vi "JsonToSteps.vi"(8 "error in":errorcluster, 11 "JSON String":string) -> (0 "error out":errorcluster, 2 "All items found?":bool, 3 "Steps":refnum<class "Step.lvclass">[](array[class]))   [LabVIEW 2023, in "Easy.SequenceManagerLabVIEW.lvlib" / "Step.lvclass"]
uses:
  Step.lvclass
  6cf8f237-96dc-4f1f-a660-aec153e8deb5.vi
  054594f7-ea92-4a54-9fad-94293ff1125a.vi
  ec343c40-536c-461c-8d01-e8b2dd1d68f3.vi
  695f3286-a13c-467f-b6c6-973f5bd1729f.vi
  <vilib>/JDP Science/JSONtext/Find Item.vi
  <vilib>/JDP Science/JSONtext/Next JSON Value.vi
  <vilib>/JDP Science/JSONtext/String Subset.vi
  <vilib>/JDP Science/JSONtext/Parsing/Advance past next JSON Value (inlined COPY).vi
  <vilib>/JDP Science/JSONtext/Parsing/Advance past whitespace.vi
  <vilib>/JDP Science/JSONtext/Parsing/Advance past String.vi
  <vilib>/JDP Science/JSONtext/Parsing/Advance past Number.vi
  <vilib>/JDP Science/JSONtext/Parsing/Advance past Line Ending.vi
  <vilib>/JDP Science/JSONtext/Parsing/Parse Full Path or Item Name.vi
  <vilib>/JDP Science/JSONtext/Parsing/Advance past Array.vi
  <vilib>/JDP Science/JSONtext/Parsing/Advance past Object.vi
  <vilib>/JDP Science/JSONtext/support/Error Cluster From Code.vi
  <vilib>/JDP Science/JSONtext/Offset/Find Item Locations by Path.vi
  <vilib>/JDP Science/JSONtext/JSON text to Variant.vi
  <vilib>/JDP Science/JSONtext/LVClass Serializer/JSONtext LVClass Serializer.lvclass
  <vilib>/JDP Science/JSONtext/JSONtext.lvlib
  Parameter/Parameter.lvclass
panel:
  # "Connector Pane"
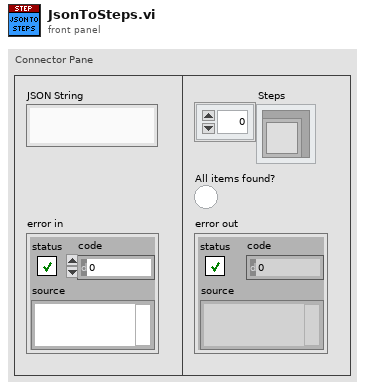
[diagram p1: front panel]
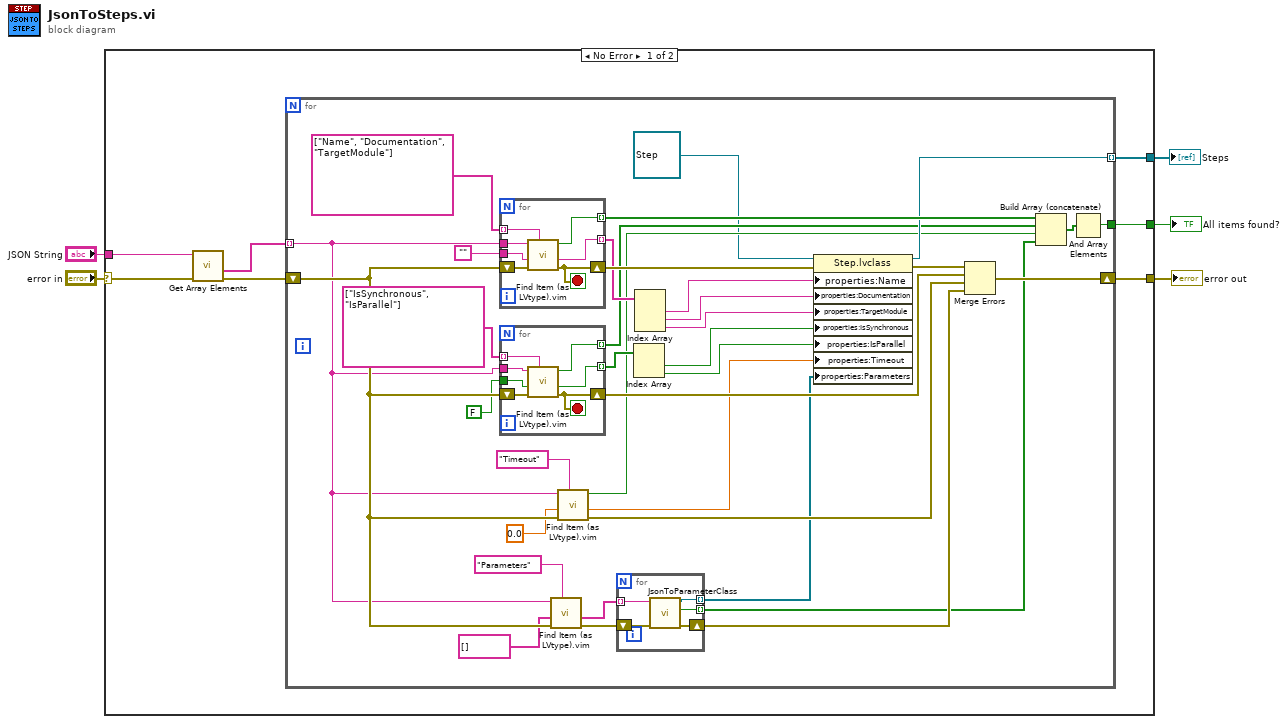
[diagram p0: block diagram]
diagram:
  n1 = case shown="No Error" "error in" {
    selector: "error in" -> [w12 w67]
    tunnel: [w10 w67] -> w4
    tunnel: "JSON String" -> [w9 _]
    tunnel: [w7 _] -> w2
    tunnel: [w6 _] -> w1
    frame No Error {
      n2 = call <vilib>:"Get Array Elements.vi"("error in (no error)"=w12, "JSON"=w9) -> ("error out"=w11:errorcluster, "<JSON>"=w8:string[])  [unwired: 7 in, 1 out]
      n3 = for {
        tunnel: w8 -> [w22] mode=indexing
        tunnel: [w18] -> w7 mode=indexing
        shift-right: [w40] -> w10
        shift-left: w11 -> [w44]
        tunnel: [w15] -> w6
        n4 = for {
          tunnel: string[] ["Name", "Documentation", "TargetModule"] -> [w64] mode=indexing
          tunnel: "" -> [w63]
          tunnel: w22 -> [w62]
          shift-right: [w65] -> w47
          shift-left: w44 -> [w66]
          tunnel: [w61] -> w35 mode=indexing
          tunnel: [w60] -> w37 mode=indexing
          stop <- w65 stop-if-true
          n5 = call "Find Item (as LVtype).vim"("$Path or Item Name"=w64, "error in (no error)"=w66, "Data Type and Default Value"=w63, "JSON"=w62) -> ("error out"=w65:errorcluster, "Data"=w61:string, "Found"=w60:bool)  [unwired: 4 in, 1 out]
        }
        n6 = for {
          tunnel: string[] ["IsSynchronous", "IsParallel"] -> [w57] mode=indexing
          tunnel: FALSE -> [w56]
          tunnel: w22 -> [w55]
          shift-right: [w58] -> w43
          shift-left: w44 -> [w59]
          tunnel: [w54] -> w29 mode=indexing
          tunnel: [w53] -> w17 mode=indexing
          stop <- w58 stop-if-true
          n7 = call "Find Item (as LVtype).vim"("$Path or Item Name"=w57, "error in (no error)"=w59, "Data Type and Default Value"=w56, "JSON"=w55) -> ("error out"=w58:errorcluster, "Data"=w54:bool, "Found"=w53:bool)  [unwired: 4 in, 1 out]
        }
        n8 = call "Find Item (as LVtype).vim"("$Path or Item Name"="Parameters", "error in (no error)"=w44, "Data Type and Default Value"=string[] [], "JSON"=w22) -> ("error out"=w46:errorcluster, "Data"=w20:string[])  [unwired: 4 in, 2 out]
        n9 = call "Find Item (as LVtype).vim"("$Path or Item Name"="Timeout", "error in (no error)"=w44, "Data Type and Default Value"=0.0, "JSON"=w22) -> ("error out"=w42:errorcluster, "Data"=w24:dbl, "Found"=w16:bool)  [unwired: 4 in, 1 out]
        n10 = for {
          tunnel: w20 -> [w50] mode=indexing
          tunnel: [w49] -> w14 mode=indexing
          tunnel: [w48] -> w19 mode=indexing
          shift-right: [w51] -> w41
          shift-left: w46 -> [w52]
          n11 = call "JsonToParameterClass.vi"("error in"=w52, "JSON String"=w50) -> ("error out"=w51:errorcluster, "All items found?"=w49:bool, "Parameter Out"=w48:refnum<class "Parameter.lvclass">)  [unwired: 7 in]
        }
        n12 = Index Array(array=w29) -> (element #1=w28:bool, element #2=w27:bool)  [unwired: 2 in]
        n13 = Index Array(array=w35) -> (element #1=w34:string, element #2=w33:string, element #3=w32:string)  [unwired: 3 in]
        n14 = property class="Step.lvclass"(reference=refnum<class "Step.lvclass"> refnum ("Easy.SequenceManagerLabVIEW.lvlib:Step.lvclass"), error in=w47, "properties:Name"=w34, "properties:Documentation"=w33, "properties:TargetModule"=w32, "properties:IsSynchronous"=w28, "properties:IsParallel"=w27, "properties:Timeout"=w24, "properties:Parameters"=w19) -> (reference out=w18:refnum<class "Step.lvclass">, error out=w45:errorcluster)
        n15 = Merge Errors(w45, w43, w42, w41) -> (w40:errorcluster)
        n16 = Build Array (concatenate)(w37, w17, w16, w14) -> (w36:bool[])
        n17 = And Array Elements(Boolean array=w36) -> (logical AND=w15:bool)
      }
    }
    frame Error {
    }
  }
  "error out" <- w4
  "Steps" <- w2
  "All items found?" <- w1
